vi "Annotate Targets.vi"(8 "Rejected particles":T1(array[cluster]), 9 "Unpaired particles":T1(array[cluster]), 10 "Measured Targets in":T2[](array[typedef]), 11 "Refnum in":T3) -> (3 "Refnum out":T3)   [LabVIEW 2014]
uses:
  <vilib>/vision/Image Controls.llb/IMAQ Image.ctl
  Vision Tote Data.ctl
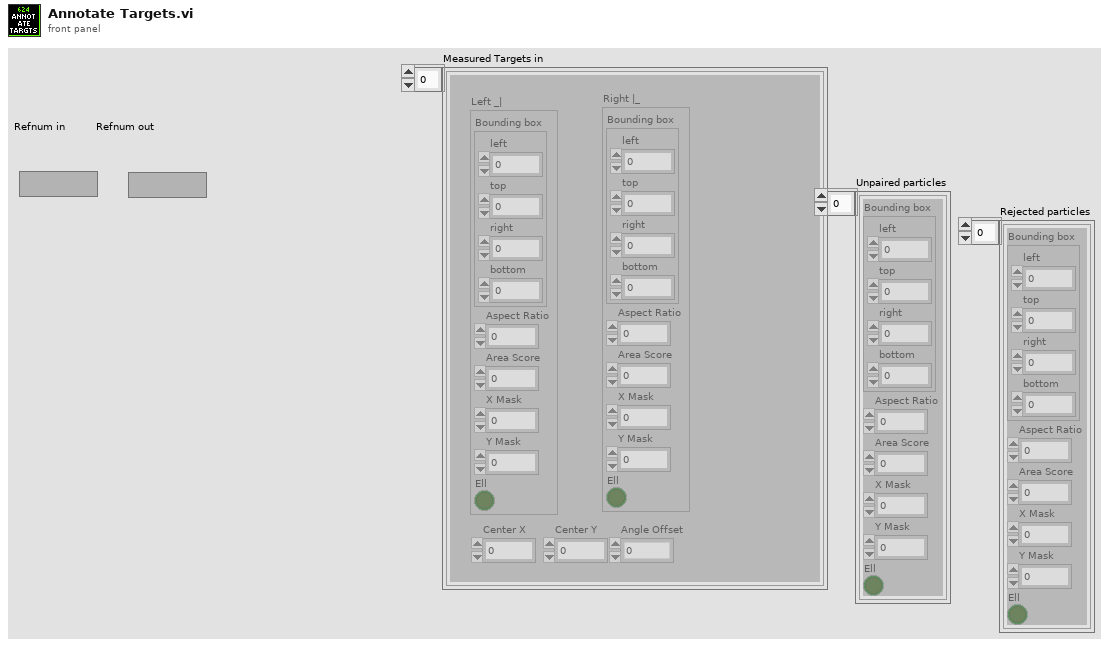
[diagram p1: front panel]
types:
  T1 = cluster{"Bounding box":cluster{"left":dbl, "top":dbl, "right":dbl, "bottom":dbl}, "Aspect Ratio":dbl, "Area Score":dbl, "X Mask":dbl, "Y Mask":dbl, "Ell":bool}[]
  T2 = typedef "Vision Tote Data.ctl" = cluster{"Left _|":cluster{"Bounding box":cluster{"left":dbl, "top":dbl, "right":dbl, "bottom":dbl}, "Aspect Ratio":dbl, "Area Score":dbl, "X Mask":dbl, "Y Mask":dbl, "Ell":bool}, "Right |_":cluster{"Bounding box":cluster{"left":dbl, "top":dbl, "right":dbl, "bottom":dbl}, "Aspect Ratio":dbl, "Area Score":dbl, "X Mask":dbl, "Y Mask":dbl, "Ell":bool}, "Center X":dbl, "Center Y":dbl, "Angle Offset":dbl}
  T3 = typedef "IMAQ Image.ctl" = refnum<image>
  T4 = typedef "Image Type" = u32
  T5 = cluster{"left":dbl, "top":dbl, "right":dbl, "bottom":dbl}
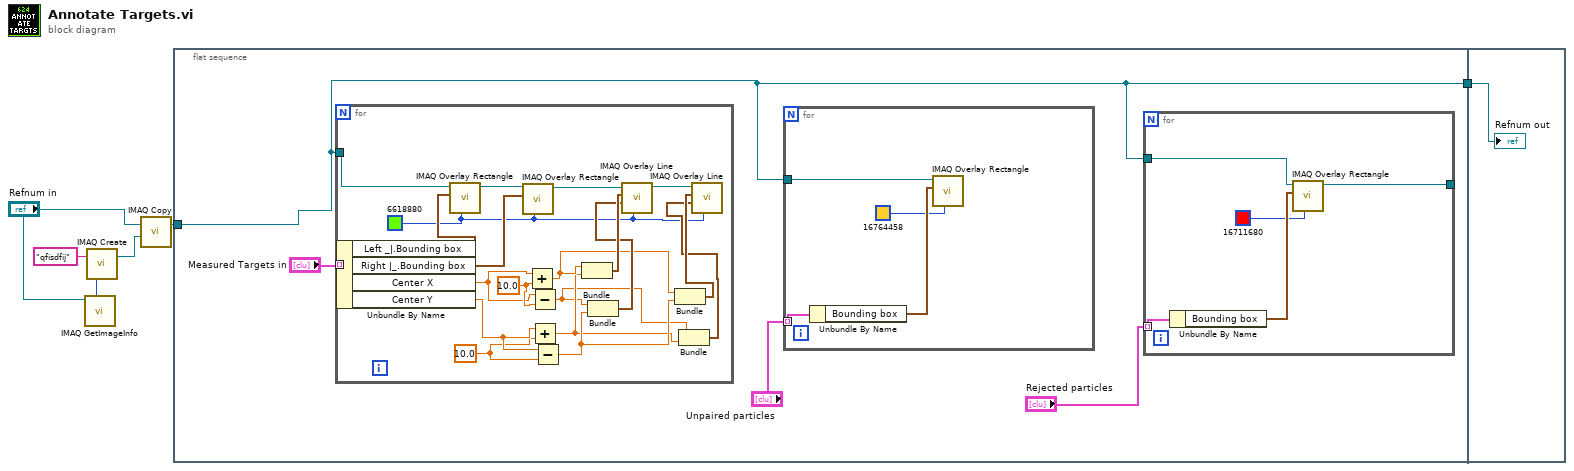
[diagram p0: block diagram]
diagram:
  n1 = call "IMAQ GetImageInfo"("Image"="Refnum in") -> ("Image Type"=w3:T4)  [unwired: 3 in, 7 out]
  n2 = call "IMAQ Create"("Image Name"="qfisdfij", "Image Type"=w3) -> ("New Image"=w5:T3)  [unwired: 3 in, 1 out]
  n3 = call "IMAQ Copy"("Image Dst"=w5, "Image Src"="Refnum in") -> ("Image Dst Out"=w2:T3)  [unwired: 4 in, 1 out]
  n4 = flat-sequence {
    tunnel: w2 -> [w7]
    tunnel: [w7] -> w1
    tunnel: w1 -> [w40]
    frame #0 {
      n5 = for {
        tunnel: w7 -> [w39]
        tunnel: "Measured Targets in" -> [w38] mode=indexing
        w29 = 10.0 ("y")
        w32 = 10.0 ("y")
        w20 = u32 6618880 ("Color")
        n6 = Unbundle By Name(w38) -> ("Left _|.Bounding box"=w37:T5, "Right |_.Bounding box"=w35:T5, "Center X"=w31:dbl, "Center Y"=w30:dbl)
        n7 = call "IMAQ Overlay Rectangle"("Color"=w20, "Rectangle"=w37, "Image"=w39) -> ("Image Out"=w36:T3)  [unwired: 7 in, 1 out]
        n8 = call "IMAQ Overlay Rectangle"("Color"=w20, "Rectangle"=w35, "Image"=w36) -> ("Image Out"=w34:T3)  [unwired: 7 in, 1 out]
        n9 = Add(x=w31, y=w32) -> (x+y=w26:dbl)
        n10 = Subtract(x=w31, y=w32) -> (x-y=w22:dbl)
        n11 = Add(x=w30, y=w29) -> (x+y=w23:dbl)
        n12 = Subtract(x=w30, y=w29) -> (x-y=w25:dbl)
        n13 = Bundle(w26, w23) -> (w28:cluster{dbl, dbl})  [unwired: 1 in]
        n14 = Bundle(w22, w25) -> (w27:cluster{dbl, dbl})  [unwired: 1 in]
        n15 = call "IMAQ Overlay Line"("Color"=w20, "End Point"=w27, "Start Point"=w28, "Image"=w34) -> ("Image Out"=w33:T3)  [unwired: 6 in, 1 out]
        n16 = Bundle(w26, w25) -> (w24:cluster{dbl, dbl})  [unwired: 1 in]
        n17 = Bundle(w22, w23) -> (w21:cluster{dbl, dbl})  [unwired: 1 in]
        n18 = call "IMAQ Overlay Line"("Color"=w20, "End Point"=w21, "Start Point"=w24, "Image"=w33) -> ()  [unwired: 6 in, 2 out]
      }
      n19 = for {
        tunnel: "Unpaired particles" -> [w19] mode=indexing
        tunnel: w7 -> [w16]
        n20 = Unbundle By Name(w19) -> ("Bounding box"=w18:T5)
        n21 = call "IMAQ Overlay Rectangle"("Color"=u32 16764458, "Rectangle"=w18, "Image"=w16) -> ()  [unwired: 7 in, 2 out]
      }
      n22 = for {
        tunnel: "Rejected particles" -> [w15] mode=indexing
        tunnel: [w14] -> _
        tunnel: w7 -> [w11]
        n23 = Unbundle By Name(w15) -> ("Bounding box"=w13:T5)
        n24 = call "IMAQ Overlay Rectangle"("Color"=u32 16711680, "Rectangle"=w13, "Image"=w11) -> ("Image Out"=w14:T3)  [unwired: 7 in, 1 out]
      }
    }
    frame #1 {
      "Refnum out" <- w40
    }
  }
